vi "GetTicVariable.vi"(5 "Address [16384=Unadressed/Global]":u16, 7 "Port Name (VISA)":refnum<visa-resource-name>, 8 "errorIn":errorcluster, 11 "Variable":string(combo)) -> (0 "errorOut":errorcluster, 1 "RawValueRead":dbl, 2 "Value":dbl, 3 "Response":string)   [LabVIEW 2021]
uses:
  VariableDescriptor.ctl
  PololuCommand.ctl
panel:
  out "VariableDescription":T1 {"Offset" format="%02x"}
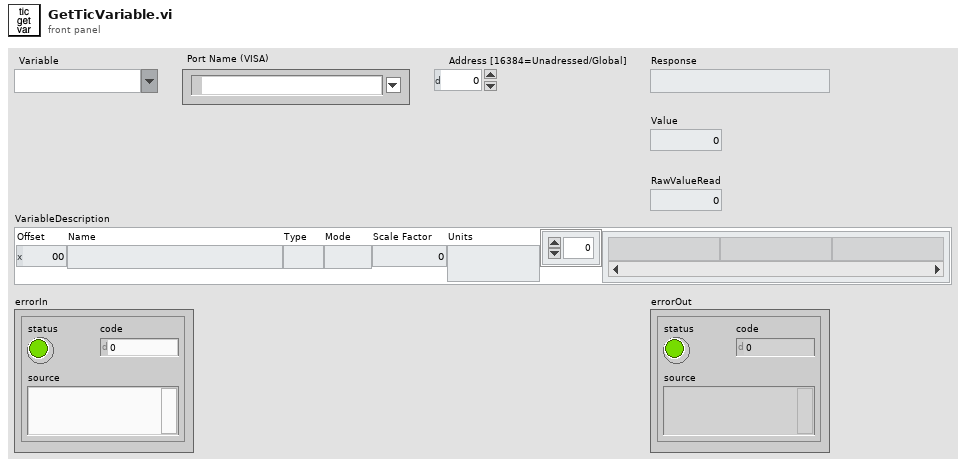
[diagram p1: front panel]
types:
  T1 = typedef "VariableDescriptor.ctl" = cluster{"Offset":u8, "Name":string, "Type":string, "Mode":string, "Scale Factor":dbl, "Units":string, "Coding":string[]}
  T2 = typedef "PololuCommand.ctl" = string
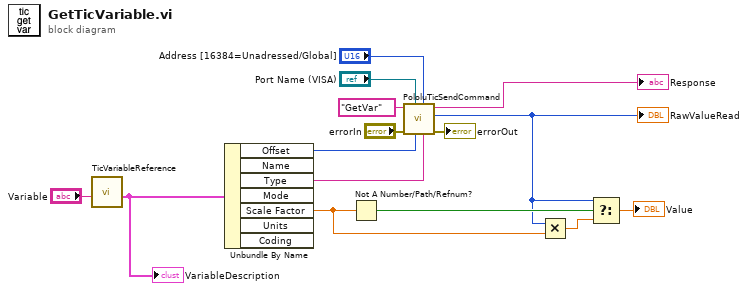
[diagram p0: block diagram]
diagram:
  n1 = call "TicVariableReference.vi"("Variable"="Variable") -> ("VariableDescription"=w13:T1)  [unwired: 9 in, 1 out]
  "VariableDescription" <- w13
  n2 = Unbundle By Name(w13) -> ("Offset"=w12:u8, "Type"=w8:string, "Scale Factor"=w4:dbl)  [unwired: 4 out]
  n3 = Not A Number/Path/Refnum?(number/path/refnum=w4) -> (NaN/Path/Refnum?=w7:bool)
  n4 = call "PololuTicSendCommand.vi"("Type"=w8, "Address"="Address [16384=Unadressed/Global]", "Register"=w12, "Port Name"="Port Name (VISA)", "errorIn"="errorIn", "PololuCommand"=T2 "GetVar") -> ("errorOut"=→"errorOut":errorcluster, "ReadValue"=w5:i64, "Response"=→"Response":string)  [unwired: 2 in, 1 out]
  "RawValueRead" <- w5
  n5 = Multiply(x=w5, y=w4) -> (x*y=w3:dbl)
  n6 = Select(t=w5, s=w7, f=w3) -> (s? t:f=→"Value":dbl)
